vi "WPI_CameraSet Image Appearance Property.vi"(8 "error in":errorcluster, 9 "Appearance":bool=TRUE, 10 "Prop String":string, 11 "address":string="192.168.0.90") -> (0 "error out":errorcluster)   [LabVIEW 2017]
doc: "This software is licensed. Open the labview\\readme\\WPI Robotics Library Open Source License.txt file for more information."
panel:
  out "For Documentation Only":string="Content-type: text/plain\n\nroot.ImageSource.I0.Sensor.WhiteBalance=auto\nroot.ImageSource.I0.Sensor.Exposure=auto\nroot.ImageSource.I0.Sensor.ExposurePriority=50\nroot.ImageSource.I0.Sensor.Brightness=60\nroot.ImageSource.I0.Sensor.ColorLevel=50\nroot.ImageSource.I0.Sensor.Sharpness=0\nroot.ImageSource.I0.Sensor.BlacklevelCorrection=0\n"
  out "Complete Response":string
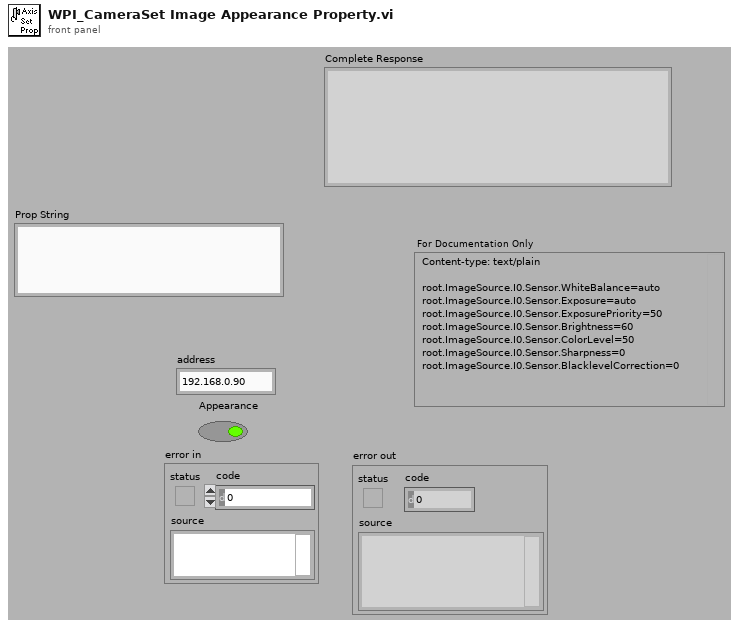
[diagram p1: front panel]
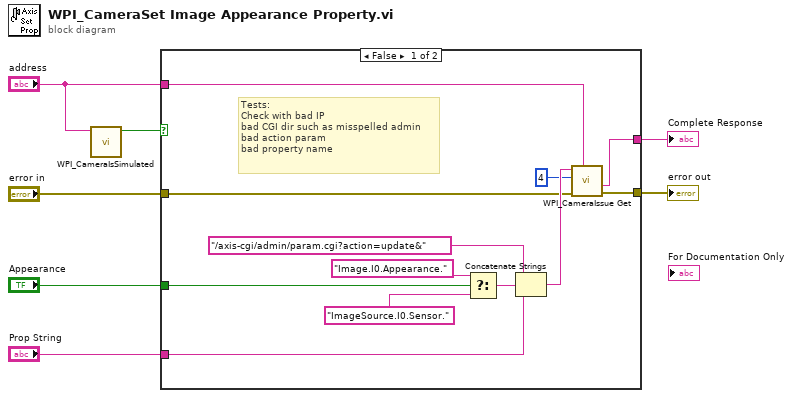
[diagram p0: block diagram]
diagram:
  n1 = call <vilib>:"WPI_CameraIsSimulated.vi"("Camera Address"="address") -> ("Simulated"=w1:bool)  [unwired: 10 in]
  n2 = case shown="False" w1 {
    tunnel: "Prop String" -> [w19 _]
    tunnel: "error in" -> [w16 w20]
    tunnel: [w15 w20] -> w5
    tunnel: [w14 _] -> w4
    tunnel: "Appearance" -> [w10 _]
    tunnel: "address" -> [w8 _]
    frame False {
      # "Tests:\nCheck with bad IP\nbad CGI dir such as misspelled admin\nbad action param\nbad property name"
      n3 = Select(t="Image.I0.Appearance.", s=w10, f="ImageSource.I0.Sensor.") -> (s? t:f=w9:string)
      n4 = Concatenate Strings("/axis-cgi/admin/param.cgi?action=update&", w9, w19) -> (w18:string)
      n5 = call <vilib>:"WPI_CameraIssue Get.vi"("address"=w8, "error in (no error)"=w16, "Number of Lines Expected"=4, "Request"=w18) -> ("error out"=w15:errorcluster, "Complete Response"=w14:string)  [unwired: 1 in, 5 out]
    }
    frame True {
      # "do nothing if simulated"
    }
  }
  "error out" <- w5
  "Complete Response" <- w4
